vi "GetWaveformByBusOrder.vi"(10 "Bus Name":string, 11 "Acq Waveforms":waveform(sgl)[](array[waveform])) -> (1 "found?":bool, 2 "Index in ABC order":i32[](array[numeric]), 3 "Bus Waveforms in ABC order":waveform(dbl)[](array[waveform]))   [LabVIEW 2017, in "McsaUtilities.lvlib"]
uses:
  <vilib>/addons/InsightCM/Utilities/MCSA/McsaUtilities.lvlib
  <vilib>/addons/InsightCM/Utilities/Analysis/MCSA/McsaAnalysisFunctions.lvlib
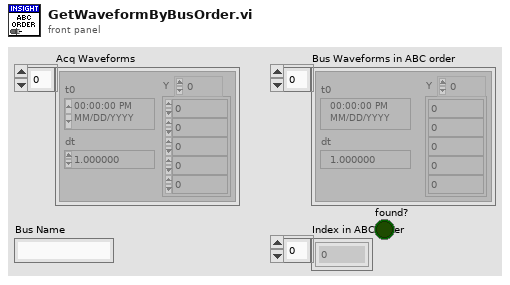
[diagram p1: front panel]
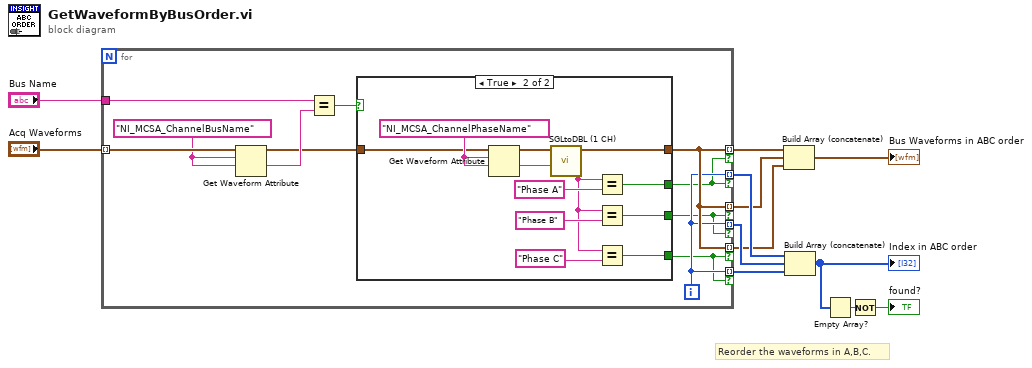
[diagram p0: block diagram]
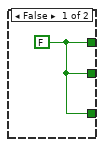
[diagram p2: hidden frame]
diagram:
  # "Reorder the waveforms in A,B,C."
  n1 = for {
    tunnel: "Acq Waveforms" -> [w23] mode=indexing
    tunnel: "Bus Name" -> [w22]
    tunnel: [w18] -> w4 mode=indexing if=w13
    tunnel: [w18] -> w5 mode=indexing if=w14
    tunnel: [w18] -> w6 mode=indexing if=w15
    tunnel: [w16] -> w10 mode=indexing if=w13
    tunnel: [w16] -> w11 mode=indexing if=w14
    tunnel: [w16] -> w12 mode=indexing if=w15
    i -> [w16]
    w21 = "NI_MCSA_ChannelBusName" ("name")
    n2 = Get Waveform Attribute(5:w21, 6:w21, 7:w23) -> (1:w20:string, 3:w19:waveform(sgl))  [unwired: 1 in, 2 out]
    n3 = Equal?(x=w22, y=w20) -> (x = y?=w17:bool)
    n4 = case shown="True" w17 {
      tunnel: w19 -> [_ w34]
      tunnel: [_ w32] -> w18
      tunnel: [w24 w27] -> w13
      tunnel: [w24 w26] -> w15
      tunnel: [w24 w25] -> w14
      frame False {
        w24 = FALSE
      }
      frame True {
        w35 = "NI_MCSA_ChannelPhaseName" ("name")
        n5 = Get Waveform Attribute(5:w35, 6:w35, 7:w34) -> (1:w29:string, 3:w33:waveform(sgl))  [unwired: 1 in, 2 out]
        n6 = call <vilib>:"SGLtoDBL (1 CH).vi"("Waveform in"=w33) -> ("Waveform out"=w32:waveform(dbl))  [unwired: 10 in]
        n7 = Equal?(x=w29, y="Phase A") -> (x = y?=w27:bool)
        n8 = Equal?(x=w29, y="Phase B") -> (x = y?=w25:bool)
        n9 = Equal?(x=w29, y="Phase C") -> (x = y?=w26:bool)
      }
    }
  }
  n10 = Build Array (concatenate)(w4, w5, w6) -> (→"Bus Waveforms in ABC order":waveform(dbl)[])
  n11 = Build Array (concatenate)(w10, w11, w12) -> (w3:i32[])
  "Index in ABC order" <- w3
  n12 = Empty Array?(array=w3) -> (empty?=w2:bool)
  n13 = Not(x=w2) -> (.not. x?=→"found?":bool)
